vi "AdvancedWriteData.vi"(9 "Data String":string, 10 "File Connection":refnum<file>) -> (1 "Sucessful?":bool, 2 "File Connection Out":refnum<file>)   [LabVIEW 2021]
uses:
  <vilib>/Utility/error.llb/DialogType.ctl
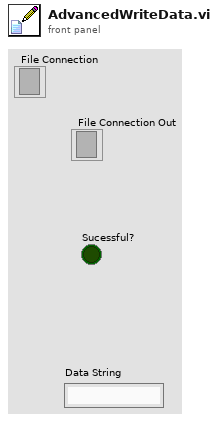
[diagram p1: front panel]
types:
  T1 = enum16{" 0 - write pressure", "1 - close then reopen file on google drive ", "2 - close reopened file on google drive open file on local drive", "3 - close file on local drive and stop"}
  T2 = enum16{"open", "replace", "create", "open or create", "replace or create", "replace or create with confirmation"}
  T3 = typedef "DialogType.ctl" = u16
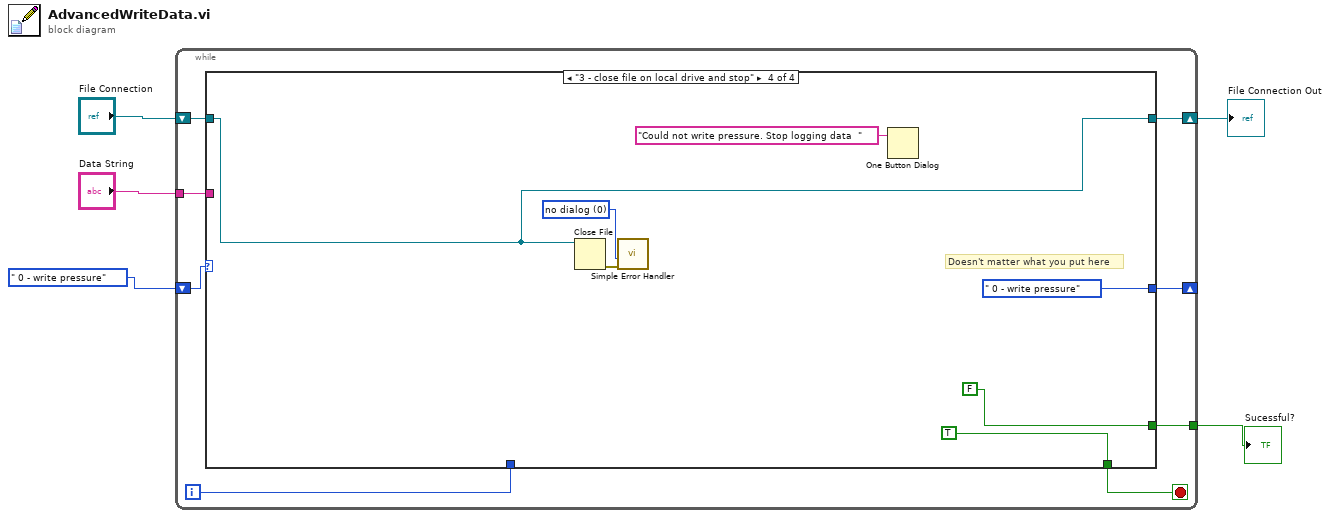
[diagram p0: block diagram]
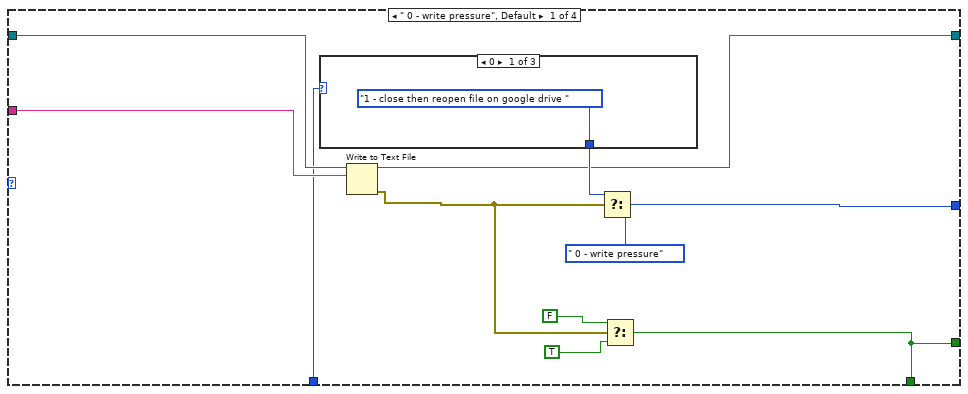
[diagram p2: hidden frame]
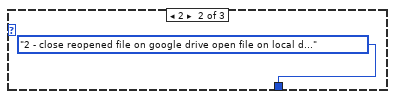
[diagram p3: hidden frame]
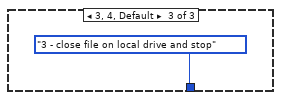
[diagram p4: hidden frame]
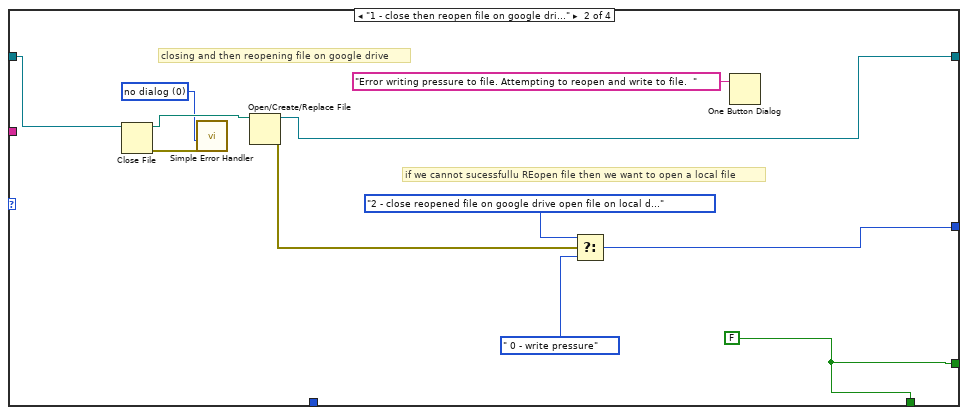
[diagram p5: hidden frame]
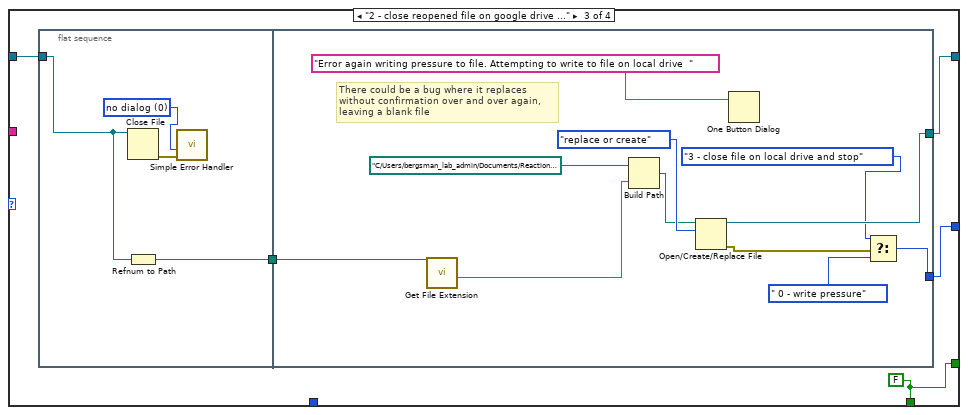
[diagram p6: hidden frame]
diagram:
  n1 = while {
    tunnel: "Data String" -> [w12]
    shift-right: [w10] -> w1
    shift-left: "File Connection" -> [w11]
    shift-right: [w9] -> _
    shift-left: T1." 0 - write pressure" -> [w13]
    tunnel: [w7] -> w2
    i -> [w6]
    stop <- w8 stop-if-true
    n2 = case shown="\"3 - close file on local drive and stop\"" w13 {
      tunnel: w12 -> [w19 _ _ _]
      tunnel: w11 -> [w18 w31 w43 w59]
      tunnel: [w17 w30 w40 w59] -> w10
      tunnel: [w16 w29 w39 T1." 0 - write pressure"] -> w9
      tunnel: [w15 w28 w41 TRUE] -> w8
      tunnel: [w15 w28 w41 FALSE] -> w7
      tunnel: w6 -> [w14 _ _ _]
      frame " 0 - write pressure", Default {
        n3 = case shown="0" w14 {
          tunnel: [T1."1 - close then reopen file on google drive " T1."2 - close reopened file on google drive open file on local drive" T1."3 - close file on local drive and stop"] -> w24
          frame 0 {
          }
          frame 2 {
          }
          frame 3, 4, Default {
          }
        }
        n4 = Write to Text File(file (use dialog)=w18, text=w19) -> (refnum out=w17:refnum<file>, error out=w20:errorcluster)  [unwired: 2 in, 1 out]
        n5 = Select(t=w24, s=w20, f=T1." 0 - write pressure") -> (s? t:f=w16:T1)
        n6 = Select(t=FALSE, s=w20, f=TRUE) -> (s? t:f=w15:bool)
      }
      frame "1 - close then reopen file on google drive " {
        w28 = FALSE
        w32 = T3 0 items=["no dialog", "OK message", "continue or stop message", "OK message + warnings", "continue/stop + warnings"] ("type of dialog (OK msg:1)")
        # "closing and then reopening file on google drive"
        # "if we cannot sucessfullu REopen file then we want to open a local file"
        n7 = Close File(refnum=w31) -> (path=w34:path, error out=w33:errorcluster)  [unwired: 1 in]
        n8 = call <vilib>:"Simple Error Handler.vi"("type of dialog (OK msg:1)"=w32, "error in (no error)"=w33) -> ()  [unwired: 3 in, 5 out]
        n9 = Open/Create/Replace File(file path (use dialog)=w34) -> (refnum out=w30:refnum<file>, error out=w38:errorcluster)  [unwired: 5 in, 1 out]
        n10 = Select(t=T1."2 - close reopened file on google drive open file on local drive", s=w38, f=T1." 0 - write pressure") -> (s? t:f=w29:T1)
        n11 = One Button Dialog(message="Error writing pressure to file. Attempting to reopen and write to file.  ") -> ()  [unwired: 1 in, 1 out]
      }
      frame "2 - close reopened file on google drive open file on local drive" {
        w41 = FALSE
        n12 = flat-sequence {
          tunnel: w43 -> [w45]
          tunnel: [w44] -> w42
          tunnel: [w57] -> w40
          tunnel: [w54] -> w39
          tunnel: w42 -> [w49]
          frame #0 {
            w46 = T3 0 items=["no dialog", "OK message", "continue or stop message", "OK message + warnings", "continue/stop + warnings"] ("type of dialog (OK msg:1)")
            n13 = Close File(refnum=w45) -> (error out=w47:errorcluster)  [unwired: 1 in, 1 out]
            n14 = Refnum to Path(1:w45) -> (0:w44:path)
            n15 = call <vilib>:"Simple Error Handler.vi"("type of dialog (OK msg:1)"=w46, "error in (no error)"=w47) -> ()  [unwired: 3 in, 5 out]
          }
          frame #1 {
            # "There could be a bug where it replaces\nwithout confirmation over and over again,\nleaving a blank file"
            n16 = call <vilib>:"Get File Extension.vi"("file"=w49) -> ("filename without extension"=w48:string)  [unwired: 6 in, 4 out]
            n17 = Build Path(base path=path "C:/Users/bergsman_lab_admin/Documents/Reaction_data" ("file path (use dialog)"), name or relative path=w48) -> (appended path=w51:path)
            n18 = Open/Create/Replace File(file path (use dialog)=w51, operation (0:open)=T2."replace or create") -> (refnum out=w57:refnum<file>, error out=w50:errorcluster)  [unwired: 4 in, 1 out]
            n19 = One Button Dialog(message="Error again writing pressure to file. Attempting to write to file on local drive  ") -> ()  [unwired: 1 in, 1 out]
            n20 = Select(t=T1."3 - close file on local drive and stop", s=w50, f=T1." 0 - write pressure") -> (s? t:f=w54:T1)
          }
        }
      }
      frame "3 - close file on local drive and stop" {
        w63 = T3 0 items=["no dialog", "OK message", "continue or stop message", "OK message + warnings", "continue/stop + warnings"] ("type of dialog (OK msg:1)")
        # "Doesn't matter what you put here"
        n21 = Close File(refnum=w59) -> (error out=w64:errorcluster)  [unwired: 1 in, 1 out]
        n22 = call <vilib>:"Simple Error Handler.vi"("type of dialog (OK msg:1)"=w63, "error in (no error)"=w64) -> ()  [unwired: 3 in, 5 out]
        n23 = One Button Dialog(message="Could not write pressure. Stop logging data  ") -> ()  [unwired: 1 in, 1 out]
      }
    }
  }
  "File Connection Out" <- w1
  "Sucessful?" <- w2
